vi "Ping_IP.vi"() -> ()   [LabVIEW 2014]
panel:
  in  "timeout":i32=100
  in  "Stopp":bool
  out "Pings total":i32
  out "unsuccessful Pings":u64
  in  "hostNameOrAddress":string="127.0.0.1"
  out "Status":i32(ring) items=["Success"=0, "DestinationNetworkUnreachable"=11002, "DestinationHostUnreachable"=11003, "DestinationProhibited, DestinationProtocolUnreachable"=11004, "DestinationPortUnreachable"=11005, "NoResources"=11006, "BadOption"=11007, "HardwareError"=11008, "PacketTooBig"=11009, "TimedOut"=11010, "BadRoute"=11012, "TtlExpired"=11013, "TtlReassemblyTimeExceeded"=11014, "ParameterProblem"=11015, "SourceQuench"=11016, "BadDestination"=11018, "DestinationUnreachable"=11040, "TimeExceeded"=11041, "BadHeader"=11042, "UnrecognizedNextHeader"=11043, "IcmpError"=11044, "DestinationScopeMismatch"=11045, "Unknown"=-1]
  # "192.168.178.30"
  # "127.0.0.1"
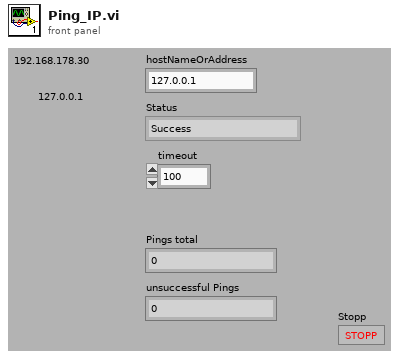
[diagram p1: front panel]
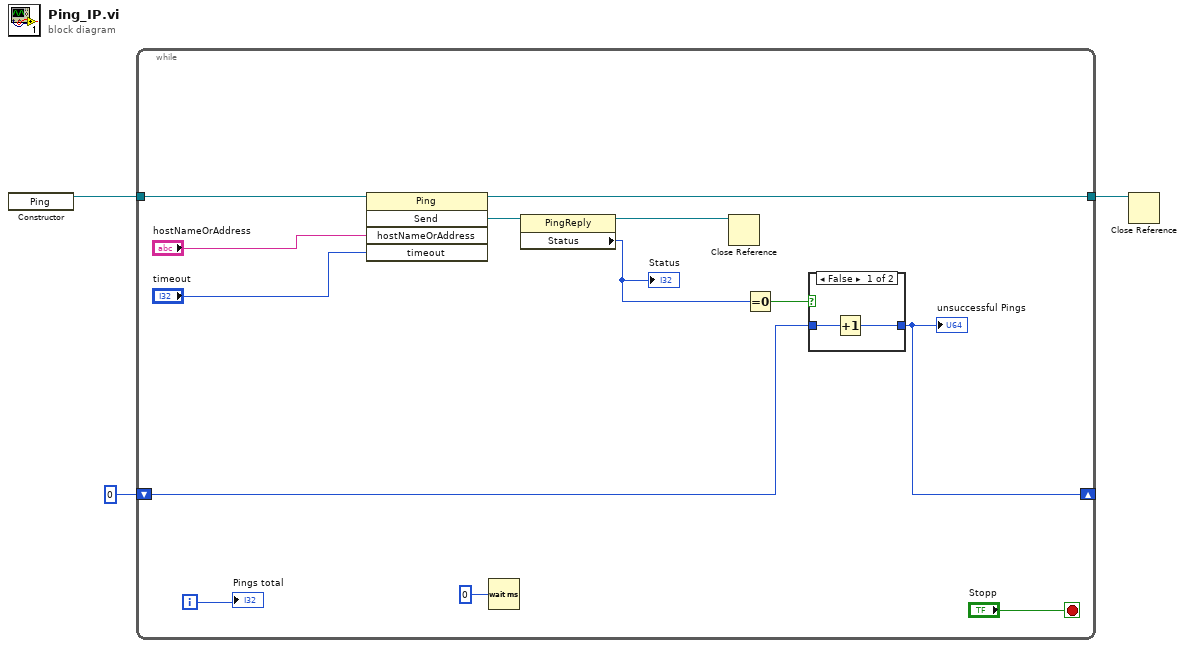
[diagram p0: block diagram]
diagram:
  n1 = constructor class="Ping"() -> (reference out=w2:refnum<k24>)  [unwired: 3 in, 2 out]
  n2 = while {
    shift-right: [w8] -> _
    shift-left: u64 0 -> [w11]
    tunnel: w2 -> [w6]
    tunnel: [w5] -> w1
    i -> [w13]
    stop <- "Stopp" stop-if-true
    n3 = invoke class="Ping" method="Send"(reference=w6, "hostNameOrAddress"="hostNameOrAddress", "timeout"="timeout") -> (reference out=w5:refnum<k24>, "Send"=w15:refnum<k24>)  [unwired: 2 in, 3 out]
    n4 = Wait (ms)(milliseconds to wait=u32 0 ("Zu wartende ms")) -> ()  [unwired: 1 out]
    n5 = property class="PingReply"(reference=w15) -> (reference out=w4:refnum<k24>, "Status"=w12:i32)  [unwired: 1 in, 1 out]
    "Status" <- w12
    n6 = Close Reference(reference=w4) -> ()  [unwired: 1 in, 1 out]
    n7 = Equal To 0?(x=w12) -> (x = 0?=w10:bool)
    n8 = case shown="False" w10 {
      tunnel: w11 -> [w18 w19]
      tunnel: [w17 w19] -> w8
      frame False {
        n9 = Increment(x=w18) -> (x+1=w17:u64)
      }
      frame True {
      }
    }
    "unsuccessful Pings" <- w8
    "Pings total" <- w13
  }
  n10 = Close Reference(reference=w1) -> ()  [unwired: 1 in, 1 out]
